vi "NT Update ValueListeners.vi"(8 "Rm Topics":string[](array[string]), 9 "New Topics":string[](array[string]), 10 "handles":cluster{"poller":u32, "topicListener":u32}) -> (0 "error out":errorcluster)   [LabVIEW 2025]
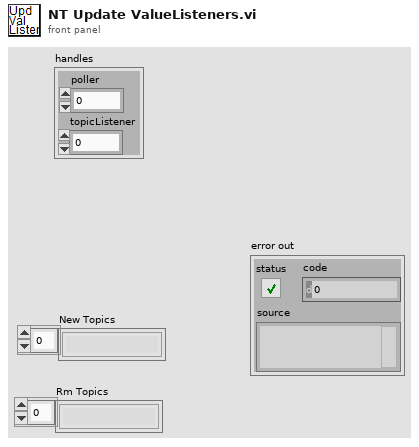
[diagram p1: front panel]
types:
  T1 = cluster{"name":string, "type":u32, "topic":u32}[]
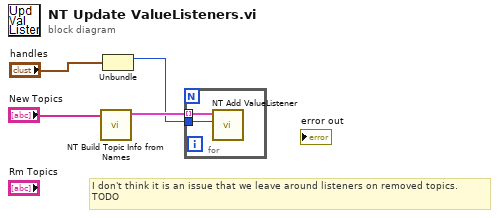
[diagram p0: block diagram]
diagram:
  # "I don't think it is an issue that we leave around listeners on removed topics. \nTODO"
  n1 = call <vilib>:"NT Build Topic Info from Names.vi"("NT Topics"="New Topics") -> ("Topic Info"=w2:T1)  [unwired: 10 in]
  n2 = Unbundle("handles") -> ("poller"=w1:u32)  [unwired: 1 out]
  n3 = for {
    tunnel: w1 -> [w6]
    tunnel: w2 -> [w5] mode=indexing
    n4 = call <vilib>:"NT Add ValueListener.vi"("poller in"=w6, "listener info"=w5) -> ()  [unwired: 8 in, 2 out]
  }
